vi "apply.vi"(8 "error in (no error)":errorcluster, 11 "BMC in":refnum<class "BMC.lvclass">) -> (0 "error out":errorcluster, 3 "BMC out":refnum<class "BMC.lvclass">)   [LabVIEW 2012, in "BMC.lvclass"]
uses:
  BMC.lvclass
  Controls/Mapping Data.ctl
panel:
  out "Mapping Data":T1
  out "DM Voltage Map":dbl[][](graph)
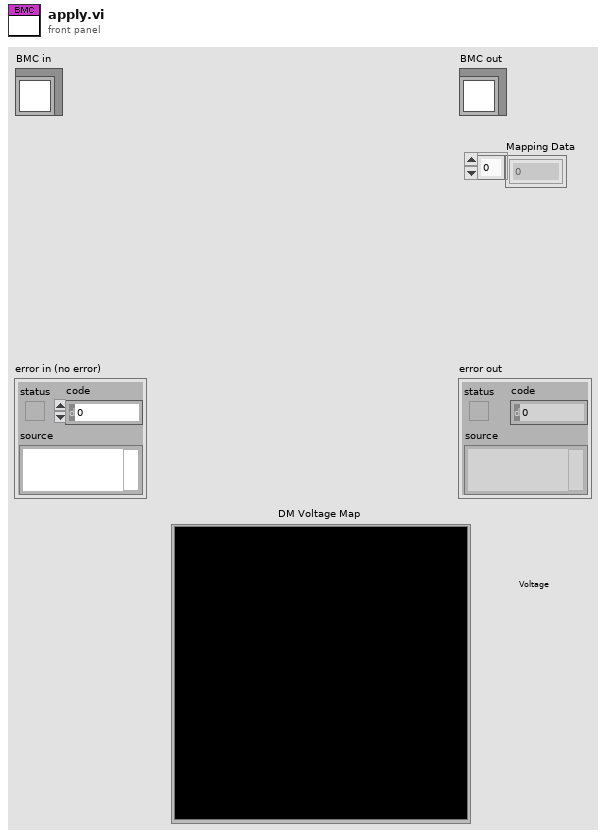
[diagram p1: front panel]
types:
  T1 = typedef "Mapping Data.ctl" = i16[]
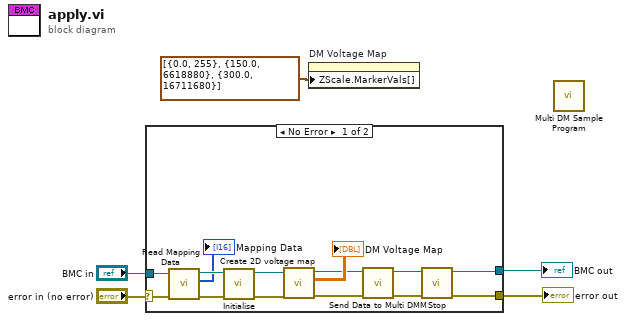
[diagram p0: block diagram]
diagram:
  n1 = case shown="No Error" "error in (no error)" {
    selector: "error in (no error)" -> [w19 w21]
    tunnel: [w10 w21] -> w4
    tunnel: [w7 w20] -> w2
    tunnel: "BMC in" -> [w15 w20]
    frame No Error {
      n2 = call-dynamic "Read Mapping Data.vi"("error in (no error)"=w19, "BMC in"=w15) -> ("error out"=w18:errorcluster, "Mapping Data"=→"Mapping Data":T1, "BMC out"=w14:refnum<class "BMC.lvclass">)  [unwired: 7 in]
      n3 = call-dynamic "Initialise.vi"("error in (no error)"=w18, "BMC in"=w14) -> ("error out"=w17:errorcluster, "BMC out"=w13:refnum<class "BMC.lvclass">)  [unwired: 8 in]
      n4 = call-dynamic "Create 2D voltage map.vi"("error in (no error)"=w17, "BMC in"=w13) -> ("error out"=w12:errorcluster, "2D Voltage Map"=→"DM Voltage Map":dbl[][], "BMC out"=w9:refnum<class "BMC.lvclass">)  [unwired: 7 in]
      n5 = call-dynamic "Send Data to Multi DMM.vi"("error in (no error)"=w12, "BMC in"=w9) -> ("error out"=w11:errorcluster, "BMC out"=w8:refnum<class "BMC.lvclass">)  [unwired: 8 in]
      n6 = call-dynamic "Stop.vi"("error in (no error)"=w11, "BMC in"=w8) -> ("error out"=w10:errorcluster, "BMC out"=w7:refnum<class "BMC.lvclass">)  [unwired: 8 in]
    }
    frame Error {
    }
  }
  "error out" <- w4
  "BMC out" <- w2
  n7 = property on="DM Voltage Map" class="IntGraph (strict)"("ZScale.MarkerVals[]"=cluster{dbl, u32}[] [{0.0, 255}, {150.0, 6618880}, {300.0, 16711680}] ("Z Scale.Marker Values[]")) -> ()  [unwired: 2 in, 2 out]
  n8 = call <userlib>:"Multi DM Sample Program.vi"() -> ()  [unwired: 1 in]
